vi "QDServGlobal.vi"() -> ()   [LabVIEW 2013]
panel:
  in  "Rate (K/min)":dbl=20.0
  in  "Target Temp":dbl=300.0
  in  "Mode":enum16{"Persistent", "Driven"}(ring)
  in  "Rate (Oe/s)":dbl=10.0
  in  "Target Field":dbl
  in  "Set Temp?":bool
  in  "Set Field?":bool
  in  "Temp Approach":enum16{"FastSettle", "NoOvershoot"}(ring)
  in  "DR Field":dbl=-0.014
  in  "DR Temperature":dbl=300.0057
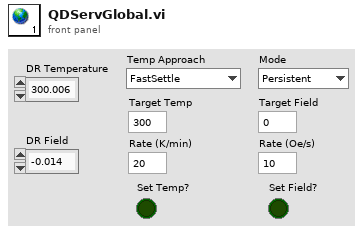
[diagram p1: front panel]
diagram:
